vi "Compute Chirp Parameters-Core.vi"(10 "AOL_Globals":T2={"Imaging Protocol"=enum."AOL Z-Stack", "Number of POI"=0, "Number of Miniscans"=0, "Number of Trials"=0, "Number of Cycles "=0, "# Averaged Frames"=0, "Laser power (%)"=0, "Pockels"=0.0, "Acquisition Length (sec)"=0.0, "Fill time (us)"=0.0, "POI Dwell time (us)"=0.0, "Miniscan Dwell time per pixel (us)"=0.0, "PMT 1"=0.0, "PMT 2"=0.0, "Back Apperture"=0.0, "Frame Size"=0, "Center Frequency"=0.0, "Field of View"=0.0, "DwellTime (us)"=0.0, "Wavelength (nm)"=0.0, "Zoom"=0.0, "AOL Z"=0.0, "AOL Mode"=enum."Raster", "GridXY"=0.0, "GridZ"=0.0, "TriggerPeriod (sec)"=0.0, "Number of Pixels in Miniscan"=0, "Experiment folder path"=path "", "X centre"=0.0, "Y centre"=0.0, "Angle (degrees)"=0.0, "Plane Mode"=0, "Threshold"=[], "Regenerate Chirps"=FALSE, "Rectangle ROI length (pixels)"=0, "Rectangle ROI height (pixels)"=0, "AOD fill"=0, "Samples Wait after Trigger"=0, "StartUp Delay"=0, "Slip Cycle"=163840, "Add Cycle"=FALSE} {"Plane Mode" items=["XY Plane"]; "Frame Size" items=["100X100"=100, "128X128"=128, "200X200"=200, "256X256"=256, "512X512"=512, "1024x1024"=1024, "2048x2048"=2048]; "Back Apperture" format="%#.6g"; "Pockels" format="%#.6g"; "PMT 2" format="%#.6g"; "PMT 1" format="%#.6g"; "Angle (degrees)" format="%#.6g"; "POI Dwell time (us)" format="%#.6g"}, 11 "Chirp in":cluster{"HexPackets":string[]}) -> (0 "error out":errorcluster, 1 "Z-stack chirp parameters":cluster{"HexPackets":string[]}[](array[cluster]), 2 "# of Z-planes":i32, 3 "Chirp out":cluster{"HexPackets":string[]})   [LabVIEW 2013]
uses:
  Typedefs/Controls/AOL_Globals.ctl
  Typedefs/Imaging Protocols enum.ctl
  Typedefs/Frame Size.ctl
  Typedefs/AOL modes.ctl
  Typedefs/Plane Mode.ctl
  Typedefs/ROI XY coordinates cluster.ctl
  Typedefs/Read Write Enum.ctl
  Global Variables/General Globals.vi
panel:
  out "ROI Coordinates (broken down to miniscans)":T1
  out "HexPackets":string[](array[string])
  out "AOL_Globals 2":T2={"Imaging Protocol"=enum."Live Imaging", "Number of POI"=0, "Number of Miniscans"=0, "Number of Trials"=0, "Number of Cycles "=0, "# Averaged Frames"=0, "Laser power (%)"=0, "Pockels"=0.0, "Acquisition Length (sec)"=0.0, "Fill time (us)"=0.0, "POI Dwell time (us)"=0.0, "Miniscan Dwell time per pixel (us)"=0.0, "PMT 1"=0.0, "PMT 2"=0.0, "Back Apperture"=0.0, "Frame Size"=200, "Center Frequency"=0.0, "Field of View"=0.0, "DwellTime (us)"=0.0, "Wavelength (nm)"=0.0, "Zoom"=0.0, "AOL Z"=0.0, "AOL Mode"=enum."Raster", "GridXY"=0.0, "GridZ"=0.0, "TriggerPeriod (sec)"=0.0, "Number of Pixels in Miniscan"=0, "Experiment folder path"=path "", "X centre"=0.0, "Y centre"=0.0, "Angle (degrees)"=0.0, "Plane Mode"=0, "Threshold"=[], "Regenerate Chirps"=FALSE, "Rectangle ROI length (pixels)"=0, "Rectangle ROI height (pixels)"=0, "AOD fill"=0, "Samples Wait after Trigger"=0, "StartUp Delay"=0, "Slip Cycle"=163840, "Add Cycle"=FALSE} {"Plane Mode" items=["XY Plane"]; "Frame Size" items=["100X100"=100, "128X128"=128, "200X200"=200, "256X256"=256, "512X512"=512, "1024x1024"=1024, "2048x2048"=2048]; "Back Apperture" format="%#.6g"; "Pockels" format="%#.6g"; "PMT 2" format="%#.6g"; "PMT 1" format="%#.6g"; "Angle (degrees)" format="%#.6g"; "POI Dwell time (us)" format="%#.6g"}
  out "?":i32
  out "?":i32
  out "Execution time 2":u32
  out "Execution time":u32
  out "Imaging Protocol":T3
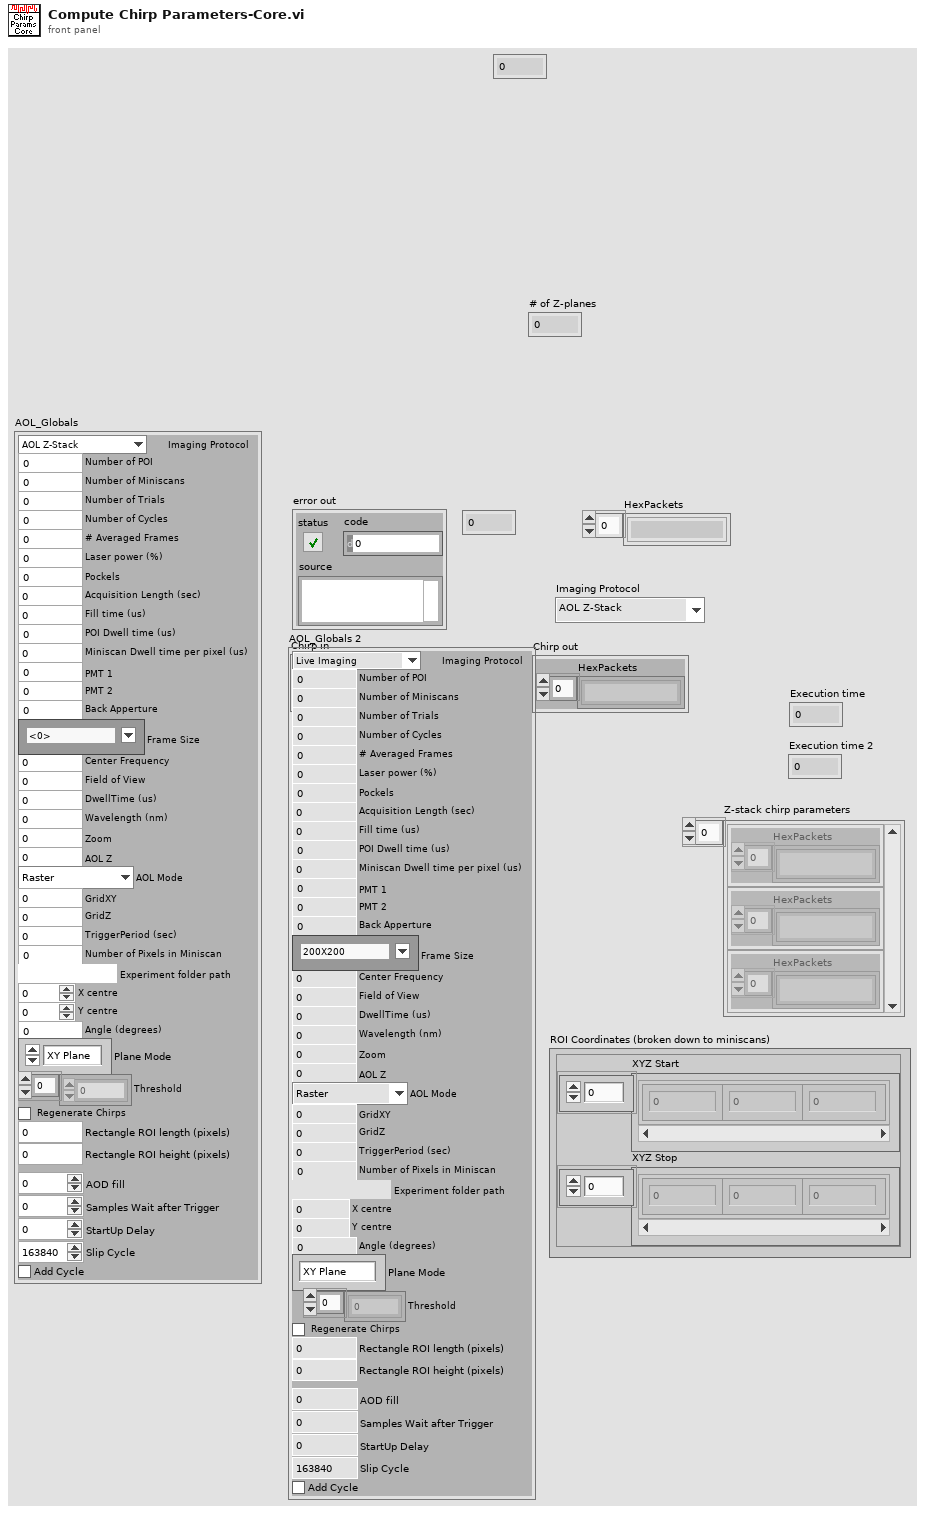
[diagram p1: front panel]
types:
  T1 = typedef "ROI XY coordinates cluster.ctl" = cluster{"XYZ Start":cluster{"X":sgl, "Y":sgl, "Z":sgl}[], "XYZ Stop":cluster{"X":sgl, "Y":sgl, "Z":sgl}[]}
  T2 = typedef "AOL_Globals.ctl" = cluster{"Imaging Protocol":T3, "Number of POI":u16, "Number of Miniscans":u16, "Number of Trials":u16, "Number of Cycles ":u64, "# Averaged Frames":u16, "Laser power (%)":u8, "Pockels":dbl, "Acquisition Length (sec)":dbl, "Fill time (us)":dbl, "POI Dwell time (us)":dbl, "Miniscan Dwell time per pixel (us)":dbl, "PMT 1":dbl, "PMT 2":dbl, "Back Apperture":dbl, "Frame Size":T4, "Center Frequency":dbl, "Field of View":dbl, "DwellTime (us)":dbl, "Wavelength (nm)":dbl, "Zoom":dbl, "AOL Z":dbl, "AOL Mode":T5, "GridXY":dbl, "GridZ":dbl, "TriggerPeriod (sec)":dbl, "Number of Pixels in Miniscan":u16, "Experiment folder path":path, "X centre":dbl, "Y centre":dbl, "Angle (degrees)":dbl, "Plane Mode":T6, "Threshold":u16[], "Regenerate Chirps":bool, "Rectangle ROI length (pixels)":u16, "Rectangle ROI height (pixels)":u16, "AOD fill":u16, "Samples Wait after Trigger":u16, "StartUp Delay":i32, "Slip Cycle":u32, "Add Cycle":bool}
  T3 = typedef "Imaging Protocols enum.ctl" = enum16{"AOL Z-Stack", "Motor Z Stack", "Functional Acquisition", "Single Plane Acquisition", "Volume Acquisition", "Live Imaging", "Live Plane Imaging", "Live Volume Imaging"}
  T4 = typedef "Frame Size.ctl" = u16
  T5 = typedef "AOL modes.ctl" = enum16{"Raster", "Structural", "Pointing", "Mini Scan", "Alignment"}
  T6 = typedef "Plane Mode.ctl" = u16
  T7 = typedef "Read Write Enum.ctl" = enum16{"Read", "Write"}
  T8 = cluster{"XYZ Start":cluster{"X":sgl, "Y":sgl, "Z":sgl}[], "XYZ Stop":cluster{"X":sgl, "Y":sgl, "Z":sgl}[]}
  T9 = typedef "ROI parameters data type.ctl" = cluster{"ROI index":dbl, "ROI ID":dbl, "ROI Time (ns)":dbl, "Pixels in ROI":dbl, "X start":dbl, "Y start":dbl, "Z start":dbl, "X stop":dbl, "Y stop":dbl, "Z stop":dbl, "Angle (deg)":dbl, "Composite ID":dbl, "Number of lines":dbl, "Frame Size":dbl, "Zoom":dbl, "Laser Power (%)":dbl, "ROI group ID":dbl}
  T10 = cluster{"M ":dbl, "Tramp":dbl[][], "A":dbl[][], "B":dbl[][], "C":dbl[][]}
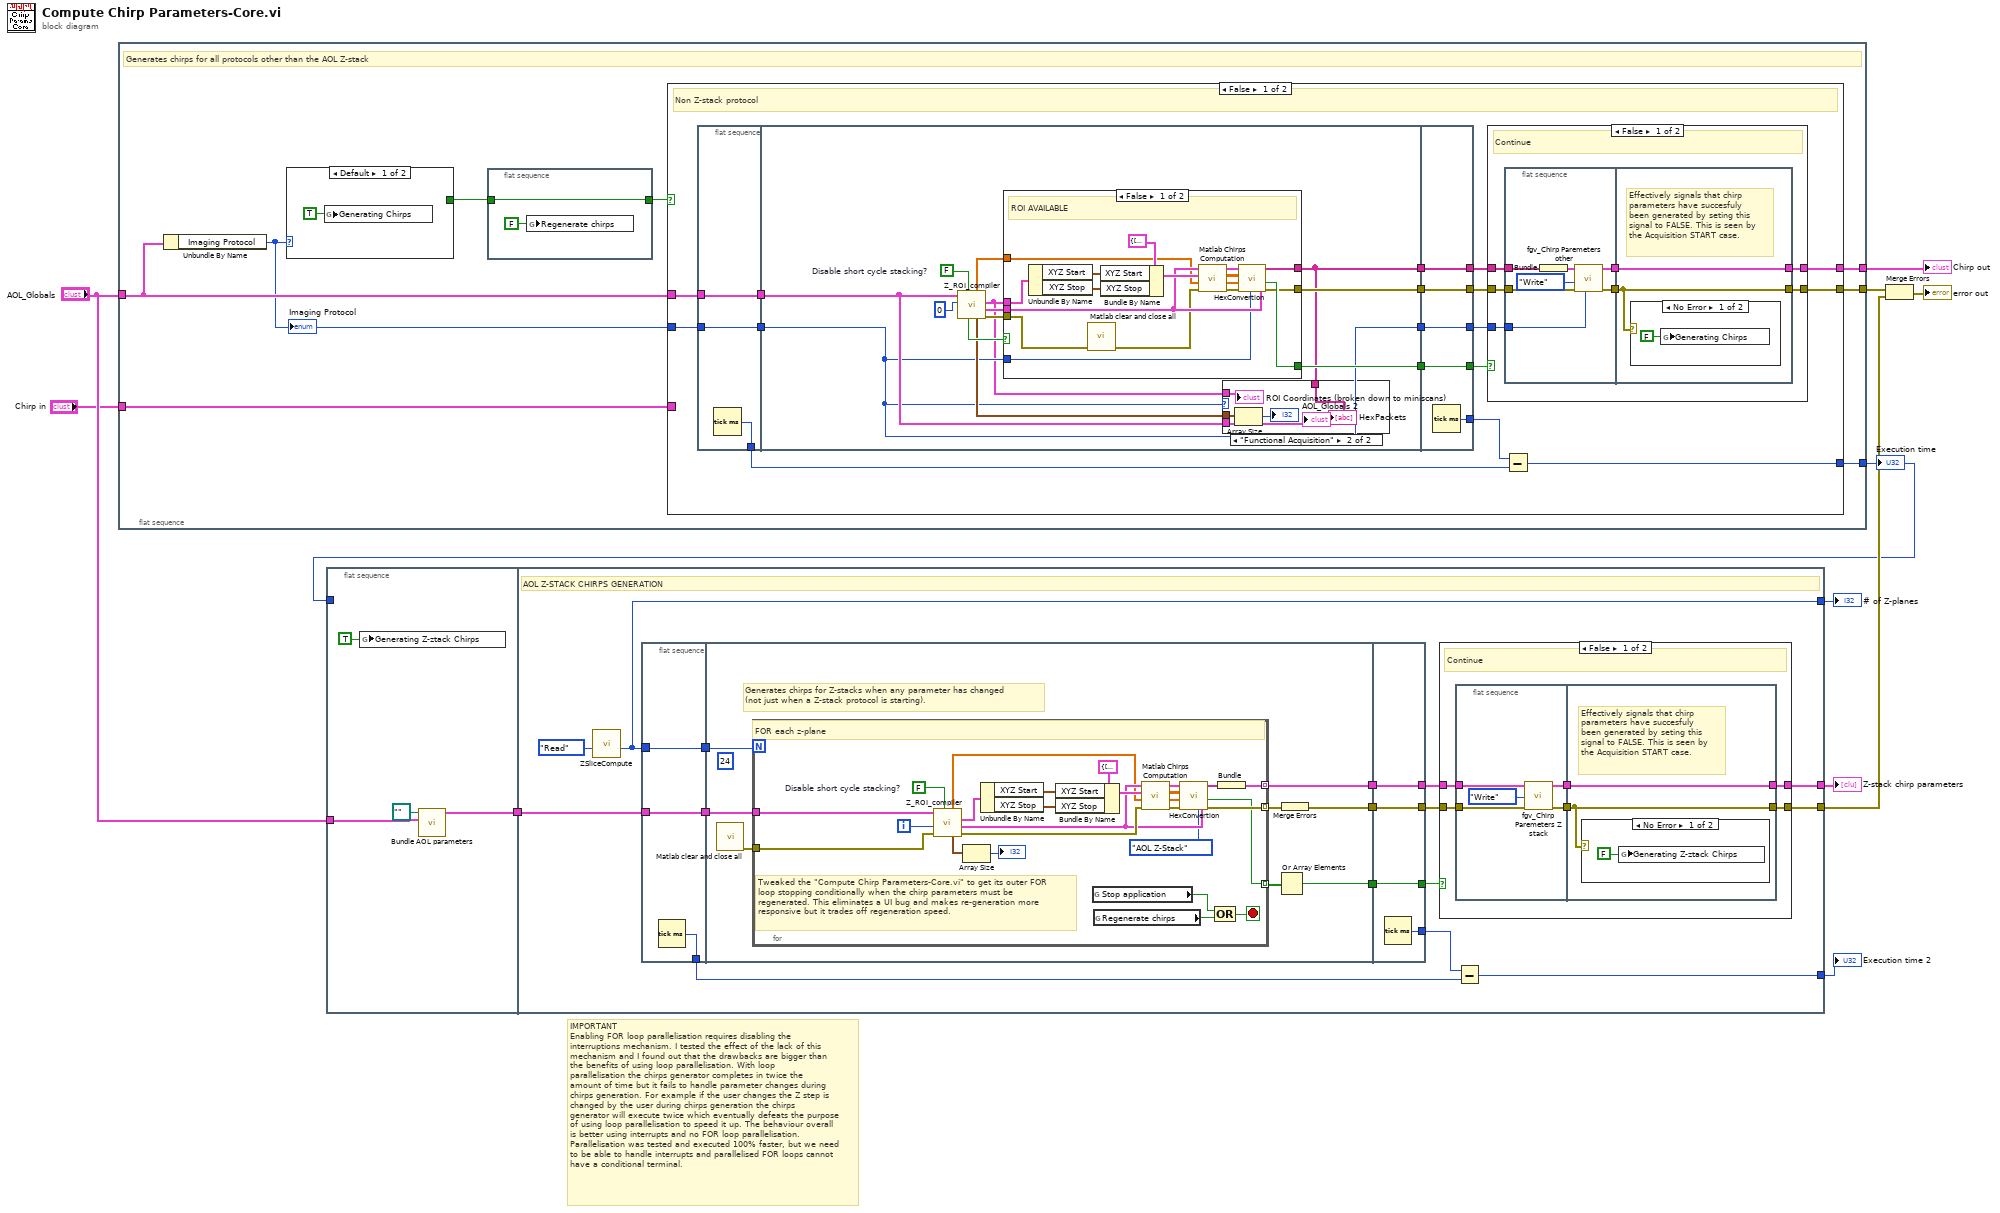
[diagram p0: block diagram]
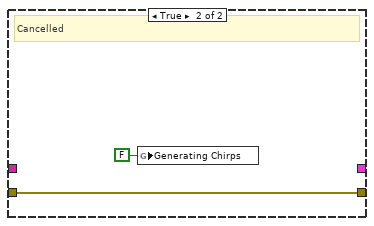
[diagram p5: hidden frame]
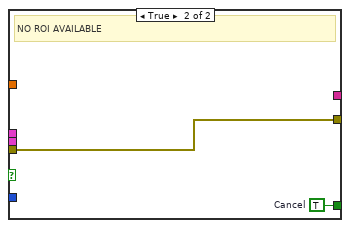
[diagram p7: hidden frame]
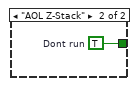
[diagram p9: hidden frame]
diagram:
  # "IMPORTANT\nEnabling FOR loop parallelisation requires disabling the interruptions mechanism. I tested the effect of the lack of this mechanism and I found out that the drawbacks are bigger than the benefits of using loop parallelisation. With loop parallelisation the chirps generator completes in twice the amount of time but it fails to handle parameter changes during chirps generation. For example if the user changes the Z step is changed by the user during chirps generation the chirps generator will execute twice which eventually defeats the purpose of using loop parallelisation to speed it up. The behaviour overall is better using interrupts and no FOR loop parallelisation. Parallelisation was tested and executed 100% faster, but we need to be able to handle interrupts and parallelised FOR loops cannot have a conditional terminal."
  n1 = flat-sequence {
    tunnel: [w19] -> w7
    tunnel: [w18] -> w2
    tunnel: [w17] -> w1
    tunnel: "AOL_Globals" -> [w16]
    tunnel: "Chirp in" -> [w15]
    frame #0 {
      # "Generates chirps for all protocols other than the AOL Z-stack"
      n2 = Unbundle By Name(w16) -> ("Imaging Protocol"=w12:T3)
      "Imaging Protocol" <- w12
      n3 = case shown="Default" w12 {
        tunnel: [_ w105] -> w14
        frame Default {
          n4 = global write "General Globals.vi" "Generating Chirps"(TRUE ("Generating Chirps")) -> ()
        }
        frame "AOL Z-Stack" {
          w105 = TRUE  # Dont run
        }
      }
      n5 = flat-sequence {
        tunnel: w14 -> [w20]
        tunnel: [w20] -> w13
        frame #0 {
          n6 = global write "General Globals.vi" "Regenerate chirps"(FALSE ("Regenerate chirps")) -> ()
        }
      }
      n7 = case shown="False" w13 {
        tunnel: [w38 w103] -> w19
        tunnel: [w37 _] -> w18
        tunnel: [w36 _] -> w17
        tunnel: w16 -> [w35 _]
        tunnel: w15 -> [_ w103]
        tunnel: w12 -> [w25 _]
        frame False {
          # "Non Z-stack protocol"
          n8 = flat-sequence {
            tunnel: w35 -> [w60]
            tunnel: [w60] -> w34
            tunnel: [w59] -> w29
            tunnel: w25 -> [w58]
            tunnel: [w58] -> w22
            tunnel: [w63] -> w33
            tunnel: [w72] -> w32
            tunnel: w34 -> [w64]
            tunnel: [w73] -> w31
            tunnel: [w62] -> w23
            tunnel: w22 -> [w62]
            tunnel: [w101] -> w27
            tunnel: [w102] -> w28
            tunnel: w33 -> [w102]
            tunnel: w32 -> [w101]
            tunnel: [w100] -> w30
            tunnel: [w99] -> w26
            tunnel: w31 -> [w99]
            tunnel: [w98] -> w24
            tunnel: w23 -> [w98]
            frame #0 {
              n9 = Tick Count (ms)() -> (millisecond timer value=w59:u32)
            }
            frame #1 {
              w66 = FALSE  # Disable short cycle stacking?
              n10 = call "Z_ROI_compiler.vi"("dISABLE"=w66, "Acquired z-plane index / volume index"=0, "AOL_Globals"=w64) -> ("error out"=w70:errorcluster, "AOL_Globals"=w69:T2, "ROI Coordinates (broken down to miniscans)"=w61:T1, "ROI Attributes (broken down to miniscans)"=w65:T9[], "Zoom"=w68:dbl[], "NO ROI AVAILABLE!!!"=w67:bool)  [unwired: 2 in, 1 out]
              n11 = case shown="False" w67 {
                tunnel: w61 -> [w95 _]
                tunnel: w70 -> [w80 w97]
                tunnel: w69 -> [w86 _]
                tunnel: w68 -> [w85 _]
                tunnel: [w84 _] -> w63
                tunnel: [w83 w96] -> w73
                tunnel: [w82 w97] -> w72
                tunnel: w62 -> [w81 _]
                frame False {
                  # "ROI AVAILABLE"
                  n12 = Unbundle By Name(w95) -> ("XYZ Start"=w92:cluster{"X":sgl, "Y":sgl, "Z":sgl}[], "XYZ Stop"=w91:cluster{"X":sgl, "Y":sgl, "Z":sgl}[])
                  n13 = call "Matlab clear and close all.vi"("error in (no error)"=w80) -> ("error out"=w79:errorcluster)  [unwired: 10 in]
                  n14 = Bundle By Name(cluster=T8 {"XYZ Start"=[{"X"=0.0, "Y"=0.0, "Z"=0.0}], "XYZ Stop"=[]} ("ROI Coordinates"), "XYZ Start"=w92, "XYZ Stop"=w91) -> (w94:T8)
                  n15 = call "Matlab Chirps Computation.vi"("error in"=w79, "Zoom"=w85, "ROI Coordinates"=w94, "AOL_Globals"=w86) -> ("error out"=w87:errorcluster, "systemVariables"=w88:dbl[], "scanVariables"=w89:dbl[][], "Chirp Parameters"=w90:T10)  [unwired: 4 in]
                  n16 = call "HexConvertion.vi"("Imaging Protocol"=w81, "AOL_Globals"=w86, "error in (no error)"=w87, "systemVariables"=w88, "scanVariables"=w89, "Chirp Parameters"=w90) -> ("error out"=w82:errorcluster, "Interrupted"=w83:bool, "HexPackets"=w84:string[])  [unwired: 3 in]
                }
                frame True {
                  w96 = TRUE  # Cancel
                  # "NO ROI AVAILABLE"
                }
              }
              n17 = case shown="\"Functional Acquisition\"" w62 {
                tunnel: w65 -> [_ w77]
                tunnel: w64 -> [_ w76]
                tunnel: w63 -> [_ w75]
                tunnel: w61 -> [_ w74]
                frame Default {
                }
                frame "Functional Acquisition" {
                  n18 = Array Size(array=w77) -> (size(s)=→"?":i32)
                  "AOL_Globals 2" <- w76
                  "HexPackets" <- w75
                  "ROI Coordinates (broken down to miniscans)" <- w74
                }
              }
            }
            frame #2 {
              n19 = Tick Count (ms)() -> (millisecond timer value=w100:u32)
            }
          }
          n20 = case shown="False" w26 {
            tunnel: [w45 _] -> w38
            tunnel: w28 -> [w44 _]
            tunnel: [w43 w57] -> w37
            tunnel: w27 -> [w42 w57]
            tunnel: w24 -> [w39 _]
            frame False {
              # "Continue"
              n21 = flat-sequence {
                tunnel: w44 -> [w52]
                tunnel: w42 -> [w49]
                tunnel: [w47] -> w41
                tunnel: [w48] -> w40
                tunnel: w39 -> [w46]
                tunnel: [w53] -> w43
                tunnel: [w54] -> w45
                tunnel: w41 -> [w54]
                tunnel: w40 -> [w53]
                frame #0 {
                  n22 = Bundle("HexPackets"=w52) -> (w51:cluster{"HexPackets":string[]})  [unwired: 1 in]
                  n23 = call "fgv_Chirp Paremeters other.vi"("Imaging Protocol in"=w46, "error in"=w49, "Function"=Read_Write_Enum."Write", "Chirps in"=w51) -> ("error out"=w48:errorcluster, "Chirps"=w47:cluster{"HexPackets":string[]})  [unwired: 5 in, 1 out]
                }
                frame #1 {
                  # "Effectively signals that chirp parameters have succesfuly been generated by seting this signal to FALSE. This is seen by the Acquisition START case."
                  n24 = case shown="No Error" w53 {
                    frame No Error {
                      n25 = global write "General Globals.vi" "Generating Chirps"(FALSE ("Generating Chirps")) -> ()
                    }
                    frame Error {
                    }
                  }
                }
              }
            }
            frame True {
              # "Cancelled"
              n26 = global write "General Globals.vi" "Generating Chirps"(FALSE ("Generating Chirps")) -> ()
            }
          }
          n27 = Subtract(x=w30, y=w29) -> (x-y=w36:u32)
        }
        frame True {
          # "Z-stack protocol"
        }
      }
    }
  }
  n28 = flat-sequence {
    tunnel: "AOL_Globals" -> [w109]
    tunnel: [w108] -> w11
    tunnel: [w106] -> _
    tunnel: w1 -> [w106]
    tunnel: w11 -> [w122]
    tunnel: [w126] -> w8
    tunnel: [w125] -> w3
    tunnel: [w124] -> w5
    tunnel: [w123] -> w9
    frame #0 {
      n29 = global write "General Globals.vi" "Generating Z-ztack Chirps"(TRUE ("Generating Chirps")) -> ()
      n30 = call "Bundle AOL parameters.vi"("AOL_Globals in"=w109, "Experiment folder path"=path "") -> ("AOL_Globals out"=w108:T2)  [unwired: 9 in]
    }
    frame #1 {
      # "AOL Z-STACK CHIRPS GENERATION"
      n31 = call "ZSliceCompute.vi"("Function"=Read_Write_Enum."Read") -> ("# of Z-planes"=w124:i32)  [unwired: 7 in, 3 out]
      n32 = flat-sequence {
        tunnel: w124 -> [w143]
        tunnel: w122 -> [w144]
        tunnel: [w144] -> w121
        tunnel: [w143] -> w120
        tunnel: [w142] -> w115
        tunnel: [w146] -> w119
        tunnel: [w150] -> w118
        tunnel: w121 -> [w152]
        tunnel: w120 -> [w149]
        tunnel: [w147] -> w117
        tunnel: [w181] -> w113
        tunnel: [w182] -> w114
        tunnel: w119 -> [w182]
        tunnel: w118 -> [w181]
        tunnel: [w180] -> w116
        tunnel: [w179] -> w112
        tunnel: w117 -> [w179]
        frame #0 {
          n33 = Tick Count (ms)() -> (millisecond timer value=w142:u32)
        }
        frame #1 {
          (unwired) 24
          # "Generates chirps for Z-stacks when any parameter has changed\n(not just when a Z-stack protocol is starting)."
          n34 = call "Matlab clear and close all.vi"() -> ("error out"=w145:errorcluster)  [unwired: 11 in]
          n35 = for {
            N: w149 -> [_]
            tunnel: [w178] -> w151 mode=indexing
            tunnel: [w177] -> w146 mode=indexing
            tunnel: w152 -> [w167]
            tunnel: [w161] -> w148 mode=indexing
            tunnel: w145 -> [w153]
            i -> [w166]
            stop <- w154 stop-if-true
            w160 = FALSE  # Disable short cycle stacking?
            # "Tweaked the \"Compute Chirp Parameters-Core.vi\" to get its outer FOR loop stopping conditionally when the chirp parameters must be regenerated. This eliminates a UI bug and makes re-generation more responsive but it trades off regeneration speed."
            # "FOR each z-plane"
            n36 = call "Z_ROI_compiler.vi"("dISABLE"=w160, "error in (no error)"=w153, "Acquired z-plane index / volume index"=w166, "AOL_Globals"=w167) -> ("error out"=w165:errorcluster, "AOL_Globals"=w164:T2, "ROI Coordinates (broken down to miniscans)"=w163:T1, "ROI Attributes (broken down to miniscans)"=w159:T9[], "Zoom"=w162:dbl[])  [unwired: 1 in, 2 out]
            n37 = Array Size(array=w159) -> (size(s)=→"?":i32)
            n38 = Unbundle By Name(w163) -> ("XYZ Start"=w173:cluster{"X":sgl, "Y":sgl, "Z":sgl}[], "XYZ Stop"=w172:cluster{"X":sgl, "Y":sgl, "Z":sgl}[])
            n39 = Bundle By Name(cluster=T8 {"XYZ Start"=[{"X"=0.0, "Y"=0.0, "Z"=0.0}], "XYZ Stop"=[]} ("ROI Coordinates"), "XYZ Start"=w173, "XYZ Stop"=w172) -> (w175:T8)
            n40 = global read "General Globals.vi" "Stop application"() -> (w155:bool)
            n41 = global read "General Globals.vi" "Regenerate chirps"() -> (w156:bool)
            n42 = call "Matlab Chirps Computation.vi"("error in"=w165, "Zoom"=w162, "ROI Coordinates"=w175, "AOL_Globals"=w164) -> ("error out"=w168:errorcluster, "systemVariables"=w169:dbl[], "scanVariables"=w170:dbl[][], "Chirp Parameters"=w171:T10)  [unwired: 4 in]
            n43 = call "HexConvertion.vi"("Imaging Protocol"=Imaging_Protocols_enum."AOL Z-Stack", "AOL_Globals"=w164, "error in (no error)"=w168, "systemVariables"=w169, "scanVariables"=w170, "Chirp Parameters"=w171) -> ("error out"=w178:errorcluster, "Interrupted"=w161:bool, "HexPackets"=w176:string[])  [unwired: 3 in]
            n44 = Compound Arithmetic op=OR(w155, w156) -> (w154:bool)
            n45 = Bundle("HexPackets"=w176) -> (w177:cluster{"HexPackets":string[]})  [unwired: 1 in]
          }
          n46 = Or Array Elements(Boolean array=w148) -> (logical OR=w147:bool)
          n47 = Merge Errors(w151) -> (w150:errorcluster)
        }
        frame #2 {
          n48 = Tick Count (ms)() -> (millisecond timer value=w180:u32)
        }
      }
      n49 = case shown="False" w112 {
        tunnel: [w132 _] -> w126
        tunnel: w114 -> [w131 _]
        tunnel: [w130 w141] -> w125
        tunnel: w113 -> [w129 w141]
        frame False {
          # "Continue"
          n50 = flat-sequence {
            tunnel: w131 -> [w135]
            tunnel: w129 -> [w133]
            tunnel: [w136] -> w128
            tunnel: [w134] -> w127
            tunnel: [w138] -> w130
            tunnel: [w139] -> w132
            tunnel: w128 -> [w139]
            tunnel: w127 -> [w138]
            frame #0 {
              n51 = call "fgv_Chirp Paremeters Z stack.vi"("error in"=w133, "Function"=Read_Write_Enum."Write", "Z-stack Chirp parameters (all Z planes) in"=w135) -> ("error out"=w134:errorcluster, "Z-stack Chirp parameters (all Z planes)"=w136:cluster{"HexPackets":string[]}[])  [unwired: 7 in]
            }
            frame #1 {
              # "Effectively signals that chirp parameters have succesfuly been generated by seting this signal to FALSE. This is seen by the Acquisition START case."
              n52 = case shown="No Error" w138 {
                frame No Error {
                  n53 = global write "General Globals.vi" "Generating Z-ztack Chirps"(FALSE ("Generating Chirps")) -> ()
                }
                frame Error {
                }
              }
            }
          }
        }
        frame True {
          # "Cancelled"
        }
      }
      n54 = Subtract(x=w116, y=w115) -> (x-y=w123:u32)
    }
  }
  n55 = Merge Errors(w2, w3) -> (→"error out":errorcluster)
  "Z-stack chirp parameters" <- w8
  "# of Z-planes" <- w5
  "Execution time" <- w1
  "Execution time 2" <- w9
  "Chirp out" <- w7
